vi "clearChannels.vi"(8 "error in":errorcluster, 11 "semaphore":T1) -> (0 "error out":errorcluster, 3 "semaphore out":T1)   [LabVIEW 2015]
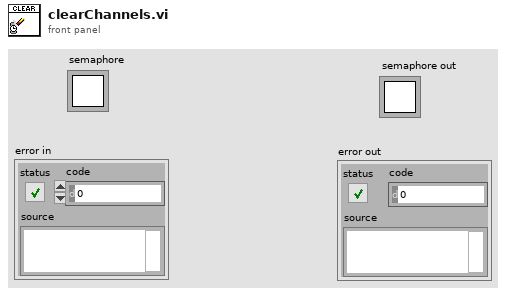
[diagram p1: front panel]
types:
  T1 = typedef "Semaphore RefNum" = refnum<k1>
  T2 = enum16{"open", "open or create", "create or replace", "create", "open (read-only)"}
  T3 = cluster{"tdms control out":refnum<k34>, "tdms historial out":refnum<k34>, "tdms sinc out":refnum<k34>}
  T4 = cluster{"tdms file out":refnum<k34>, "tdms historial out":refnum<k34>, "tdms file out":refnum<k34>}
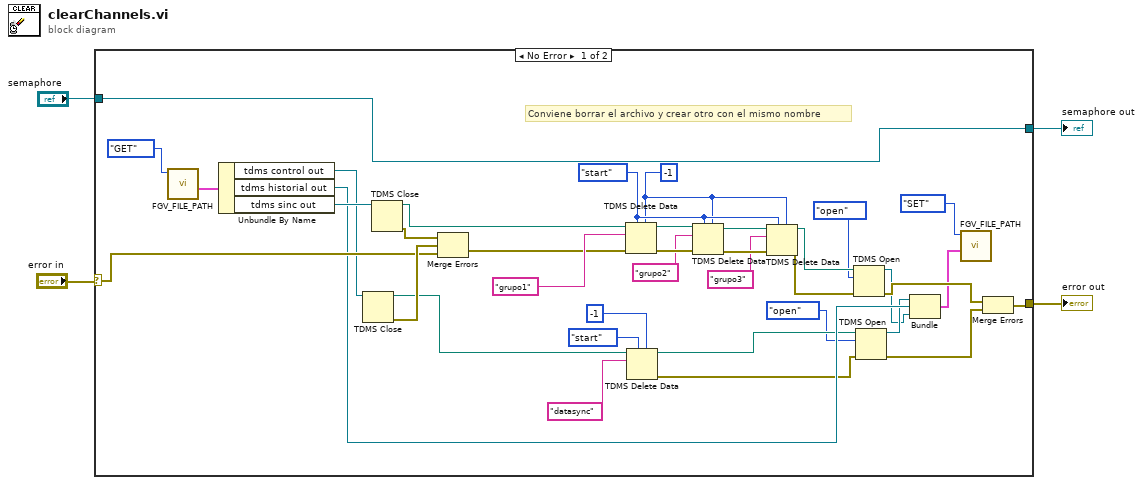
[diagram p0: block diagram]
diagram:
  n1 = case shown="No Error" "error in" {
    selector: "error in" -> [w26 w42]
    tunnel: "semaphore" -> [w30 w43]
    tunnel: [w30 w43] -> w3
    tunnel: [w14 w42] -> w2
    frame No Error {
      w34 = i64 -1 ("count (-1: all)")
      w35 = enum16{"start", "end"}."start" ("from (0: start)")
      # "Conviene borrar el archivo y crear otro con el mismo nombre"
      n2 = call "FGV_FILE_PATH.vi"("Function"=enum16{"GET", "SET"}."GET") -> ("Data Out"=w7:T3)  [unwired: 10 in]
      n3 = Unbundle By Name(w7) -> ("tdms control out"=w23:refnum<k34>, "tdms historial out"=w18:refnum<k34>, "tdms sinc out"=w24:refnum<k34>)
      n4 = TDMS Close(11:w23) -> (0:w27:errorcluster, 3:w22:path)  [unwired: 1 in]
      n5 = TDMS Close(11:w24) -> (0:w29:errorcluster, 3:w25:path)  [unwired: 1 in]
      n6 = Merge Errors(w29, w27, w26) -> (w28:errorcluster)
      n7 = TDMS Delete Data(5:w34, 7:w35, 8:w28, 10:"grupo1" ("group name in"), 11:w25) -> (0:w39:errorcluster, 3:w40:path)  [unwired: 2 in]
      n8 = TDMS Delete Data(5:i64 -1 ("count (-1: all)"), 7:enum16{"start", "end"}."start" ("from (0: start)"), 10:"datasync" ("group name in"), 11:w22) -> (0:w17:errorcluster, 3:w13:path)  [unwired: 3 in]
      n9 = TDMS Delete Data(5:w34, 7:w35, 8:w39, 10:"grupo2" ("group name in"), 11:w40) -> (0:w37:errorcluster, 3:w36:path)  [unwired: 2 in]
      n10 = TDMS Delete Data(5:w34, 7:w35, 8:w37, 10:"grupo3" ("group name in"), 11:w36) -> (0:w20:errorcluster, 3:w21:path)  [unwired: 2 in]
      n11 = TDMS Open(8:w20, 10:T2."open" ("operation (0:open)"), 11:w21) -> (0:w16:errorcluster, 3:w10:refnum<k34>)  [unwired: 4 in]
      n12 = TDMS Open(8:w17, 10:T2."open" ("operation (0:open)"), 11:w13) -> (0:w15:errorcluster, 3:w11:refnum<k34>)  [unwired: 4 in]
      n13 = Bundle("tdms file out"=w11, "tdms historial out"=w18, "tdms file out"=w10) -> (w9:T4)  [unwired: 1 in]
      n14 = call "FGV_FILE_PATH.vi"("Data In"=w9, "Function"=enum16{"GET", "SET"}."SET") -> ()  [unwired: 9 in, 1 out]
      n15 = Merge Errors(w16, w15) -> (w14:errorcluster)
    }
    frame Error {
    }
  }
  "error out" <- w2
  "semaphore out" <- w3
